vi "dfd_FXP PtByPt Lattice ARMA (one multiplier).vi"(6 "state in":i64[](array[numeric]), 7 "FXPOPs":T5[](array[typedef]) {"source" items=["Coef a/k"=0, "Coef b/v"=7, "Input"=1, "Output"=2, "Multiplicand"=3, "Product"=4, "Sum"=5, "Delay"=6, "Gain"=8]}, 8 "filtering statistics in":T4(array[cluster]) {"statistics information"."min value" format="%.2f"; "statistics information"."max value" format="%.2f"; "Quantizer Source" items=["Coefficients a/k"=0, "Coefficients b/v"=7, "Input"=1, "Output"=2, "Multiplicand"=3, "Product"=4, "Sum"=5, "Delay"=6]}, 9 "coef v[M..0]":T1, 10 "coef k[M..1]":T1, 11 "x":T7={"value"=0, "wl"=0, "iwl"=0, "Signed"=TRUE} {"value" format="%.0x"}) -> (0 "filtering statistics out":T4(array[cluster]) {"statistics information"."min value" format="%.2f"; "statistics information"."max value" format="%.2f"; "Quantizer Source" items=["Coefficients a/k"=0, "Coefficients b/v"=7, "Input"=1, "Output"=2, "Multiplicand"=3, "Product"=4, "Sum"=5, "Delay"=6]}, 3 "filtered x":T7={"value"=0, "wl"=0, "iwl"=0, "Signed"=TRUE} {"value" format="%.0x"}, 4 "state out":i64[](array[numeric]))   [LabVIEW 2017, in "NI_DigFilter_FXP.lvlib"]
uses:
  <vilib>/addons/Digital Filter Design/NI_DigFilter_FXP.lvlib
  <vilib>/addons/Digital Filter Design/_Objects.llb/dfd_DFXP Data Type (scaler).ctl
  <vilib>/addons/Digital Filter Design/_Objects.llb/dfd_DFXP Operation Parameter.ctl
  <vilib>/addons/Digital Filter Design/_Objects.llb/dfd_Internal Quantization Srcs.ctl
  <vilib>/addons/Digital Filter Design/_Objects.llb/dfd_DFXP Data Type (vector).ctl
  <vilib>/addons/Digital Filter Design/_Objects.llb/DFD Quantization Sources.ctl
  <vilib>/addons/Digital Filter Design/_Objects.llb/DFD FXP Statistics Data.ctl
  <vilib>/addons/Digital Filter Design/NI_DigFilterLicensed.lvlib
panel:
  in  "DFXP array type":T1
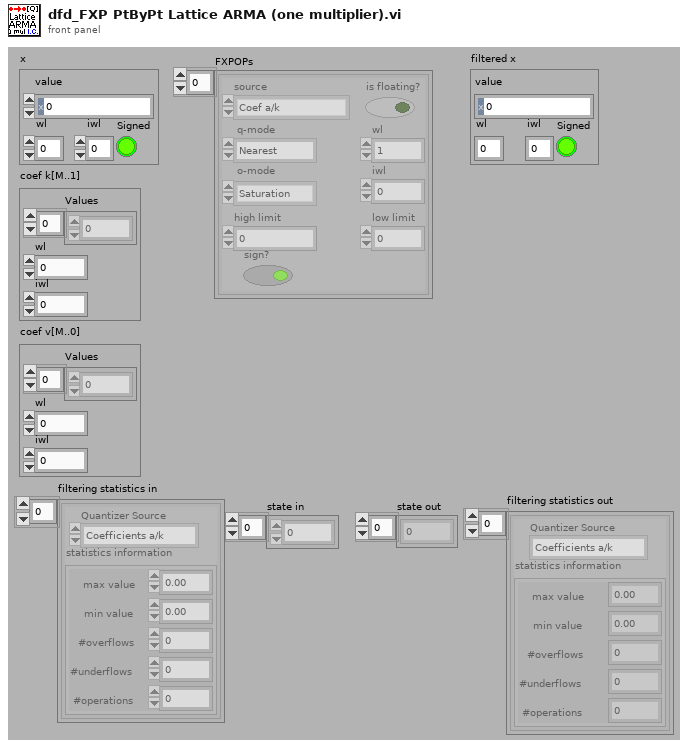
[diagram p1: front panel]
types:
  T1 = typedef "dfd_DFXP Data Type (vector).ctl" = cluster{"Values":i64[], "wl":i16, "iwl":i16}
  T2 = typedef "NI_DigFilterLicensed.lvlib/DFD Quantization Sources.ctl" = u16
  T3 = typedef "NI_DigFilterLicensed.lvlib/DFD FXP Statistics Data.ctl" = cluster{"max value":ext, "min value":ext, "#overflows":i32, "#underflows":i32, "#operations":i32}
  T4 = cluster{"Quantizer Source":T2, "statistics information":T3}[]
  T5 = typedef "dfd_DFXP Operation Parameter.ctl" = cluster{"source":T6, "is floating?":bool, "o-mode":enum16{"Saturation", "Wrap"}, "q-mode":enum16{"Nearest", "Truncation"}, "wl":i16, "high limit":i64, "low limit":i64, "iwl":i16, "sign?":bool}
  T6 = typedef "NI_DigFilterLicensed.lvlib/dfd_Internal Quantization Srcs.ctl" = u16
  T7 = typedef "dfd_DFXP Data Type (scaler).ctl" = cluster{"value":i64, "wl":i16, "iwl":i16, "Signed":bool}
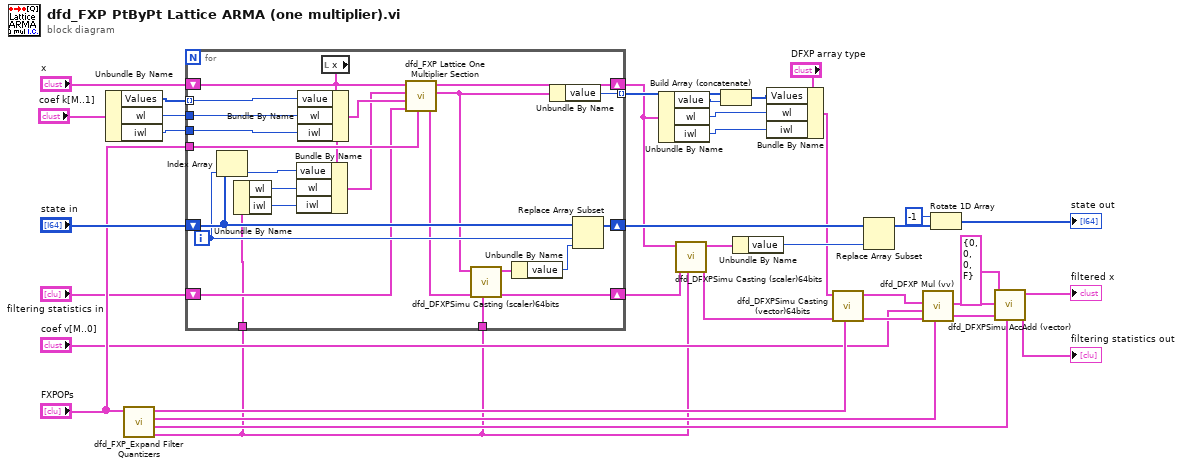
[diagram p0: block diagram]
diagram:
  n1 = Unbundle By Name("coef k[M..1]") -> ("Values"=w10:i64[], "wl"=w9:i16, "iwl"=w8:i16)
  n2 = call <vilib>:"dfd_FXP_Expand Filter Quantizers.vi"("FXPOPs"="FXPOPs") -> ("Delay"=w7:T5, "Sum"=w20:T5, "Product"=w23:T5, "Multiplicand"=w25:T5)  [unwired: 7 out]
  n3 = for {
    shift-right: [w55] -> w12
    shift-left: "x" -> [w41]
    shift-right: [w59] -> w33
    shift-left: "state in" -> [w60]
    tunnel: w7 -> [w50]
    tunnel: "FXPOPs" -> [w54]
    shift-right: [w52] -> w27
    shift-left: "filtering statistics in" -> [w53]
    tunnel: [w37] -> w26 mode=indexing
    tunnel: w10 -> [w49] mode=indexing
    tunnel: w9 -> [w45]
    tunnel: w8 -> [w44]
    tunnel: w7 -> [w40]
    i -> [w58]
    n4 = Index Array(array=w60, index=w58) -> (element=w56:i64)
    n5 = Unbundle By Name(w40) -> ("wl"=w39:i16, "iwl"=w38:i16)
    n6 = Bundle By Name(cluster=w41, "value"=w56, "wl"=w39, "iwl"=w38) -> (w42:T7)
    n7 = local read "x"() -> (w46:T7)
    n8 = Bundle By Name(cluster=w46, "value"=w49, "wl"=w45, "iwl"=w44) -> (w47:T7)
    n9 = call <vilib>:"dfd_FXP Lattice One Multiplier Section.vi"("FXPOPs"=w54, "filtering statistics in"=w53, "k(m)"=w47, "w(m-1)"=w42, "x(m)"=w41) -> ("filtering statistics out"=w51:T4, "w(m)"=w48:T7, "x(m-1)"=w55:T7)  [unwired: 1 out]
    n10 = call <vilib>:"dfd_DFXPSimu Casting (scaler)64bits.vi"("op params"=w50, "filtering statistics in"=w51, "Value in"=w48) -> ("filtering statistics out"=w52:T4, "Value out"=w57:T7)  [unwired: 2 in, 5 out]
    n11 = Unbundle By Name(w57) -> ("value"=w43:i64)
    n12 = Unbundle By Name(w48) -> ("value"=w37:i64)
    n13 = Replace Array Subset(array=w60, new element=w43, index=w58) -> (w59:i64[])
  }
  n14 = Unbundle By Name(w12) -> ("value"=w6:i64, "wl"=w2:i16, "iwl"=w1:i16)
  n15 = call <vilib>:"dfd_DFXPSimu Casting (scaler)64bits.vi"("op params"=w7, "filtering statistics in"=w27, "Value in"=w12) -> ("filtering statistics out"=w24:T4, "Value out"=w32:T7)  [unwired: 2 in, 5 out]
  n16 = Build Array (concatenate)(w26, w6) -> (w11:i64[])
  n17 = Unbundle By Name(w32) -> ("value"=w5:i64)
  n18 = Bundle By Name(cluster="DFXP array type", "Values"=w11, "wl"=w2, "iwl"=w1) -> (w4:T1)
  n19 = call <vilib>:"dfd_DFXPSimu Casting (vector)64bits.vi"("op params"=w25, "filtering statistics in"=w24, "Value in"=w4) -> ("filtering statistics out"=w17:T4, "Value out"=w16:T1)  [unwired: 1 in, 6 out]
  n20 = Replace Array Subset(array=w33, new element=w5) -> (w30:i64[])  [unwired: 1 in]
  n21 = call <vilib>:"dfd_DFXP Mul (vv).vi"("op params"=w23, "filtering statistics in"=w17, "Value in 2"="coef v[M..0]", "Value in"=w16) -> ("filtering statistics out"=w22:T4, "Value out"=w21:T1)  [unwired: 6 out]
  n22 = Rotate 1D Array(1:w30, 2:-1 ("n")) -> (0:→"state out":i64[])
  n23 = call <vilib>:"dfd_DFXPSimu AccAdd (vector).vi"("op params"=w20, "filtering statistics in"=w22, "addends"=w21, "acc in"=T7 {"value"=0, "wl"=0, "iwl"=0, "Signed"=FALSE}) -> ("filtering statistics out"=→"filtering statistics out":T4, "acc out"=→"filtered x":T7)  [unwired: 1 in, 5 out]
